vi "Table, Show All Rows.vi"(8 "error in":errorcluster, 11 "Tbl Refnum":refnum<vi>) -> (0 "error out":errorcluster, 3 "Tbl Refnum out":refnum<vi>)   [LabVIEW 2010]
doc: "Shows all table rows plus an empty row.\nSince all rows are displayed, the vertical scrollbar is hidden."
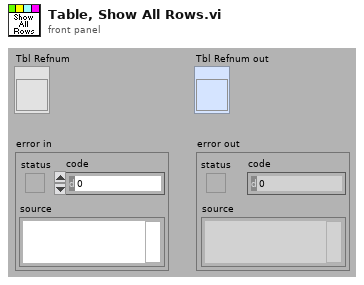
[diagram p1: front panel]
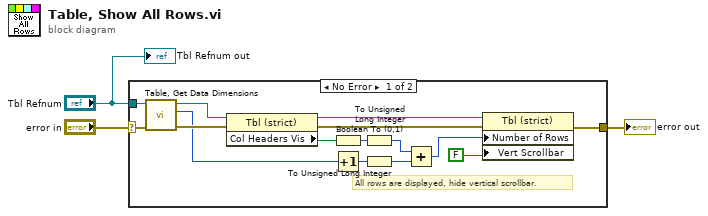
[diagram p0: block diagram]
diagram:
  n1 = case shown="No Error" "error in" {
    selector: "error in" -> [w15 w19]
    tunnel: [w10 w19] -> w3
    tunnel: "Tbl Refnum" -> [w16 _]
    frame No Error {
      # "All rows are displayed, hide vertical scrollbar."
      n2 = call "Table, Get Data Dimensions.vi"("error in"=w15, "Tbl Refnum"=w16) -> ("error out"=w18:errorcluster, "row_n"=w13:i32, "Tbl Refnum out"=w17:refnum<vi>)  [unwired: 6 in, 1 out]
      n3 = property class="Tbl (strict)"(reference=w17, error in=w18) -> (reference out=w8:refnum<vi>, error out=w11:errorcluster, "Col Headers Vis"=w14:bool)
      n4 = Boolean To (0,1)(Boolean=w14) -> (0, 1=w6:i16)
      n5 = Increment(x=w13) -> (x+1=w12:i32)
      n6 = To Unsigned Long Integer(number=w6) -> (unsigned 32bit integer=w5:u32)
      n7 = To Unsigned Long Integer(number=w12) -> (unsigned 32bit integer=w7:u32)
      n8 = Add(x=w5, y=w7) -> (x+y=w9:u32)
      n9 = property class="Tbl (strict)"(reference=w8, error in=w11, "Number of Rows"=w9, "Vert Scrollbar"=FALSE) -> (error out=w10:errorcluster)  [unwired: 1 out]
    }
    frame Error {
    }
  }
  "error out" <- w3
  "Tbl Refnum out" <- "Tbl Refnum"
